vi "IMAQController.destructor.vi"(0 "i ref in":refnum<vi>, 5 "error in (no error)":errorcluster) -> (19 "error out":errorcluster)   [LabVIEW 2014, in "IMAQController.lvlib"]
doc: "This is the destructor of a class.\n\nLicense Agreement for this software:\n\nCopyright (C)\nGesellschaft für Schwerionenforschung, GSI\nPlanckstr. 1\n64291 Darmstadt\nGermany\n\nContact: D.Beck@gsi.de \n\nThis program is free software; you can redistribute it and/or modify it under the terms of the \nGNU General Public License as published by the Free Software Foundation; either version 2 of \nthe license, or (at your option) any later version.\n\nThis program is distributed in the hope that it will be useful, but WITHOUT ANY WARRANTY; \nwithout even the implied warranty of MERCHANTABILITY or FITNESS FOR A PARTICULAR PURPOSE. See the GNU General License for more details (http://www.gnu.org).\n\nGesellschaft für Schwerionenforschung, GSI\nPlanckstr. 1, 64291 Darmstadt, Germany\nFor all questions and ideas contact: M.Richter@gsi.de, H.Brand@gsi.de or D.Beck@gsi.de.\nLast update: 16-JUN-2004"
uses:
  IMAQController.lvlib
  CSCore/CSSystem/CoreLib/CoreLib.string 2 byte array.vi
  CSCore/BaseGUI/BaseGUI.lvlib
  CSCore/BaseProcess/BaseProcess.lvlib
  CSlibraries-extern/DimLVEvent/LVDimInterface/LVDimInterface.lvlib
  CSCore/CSSystem/CSSystemLib/CSSystemLib.lvlib
  CSCore/CSSystem/CoreLib/CoreLib.lvlib
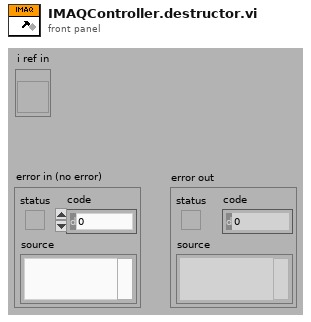
[diagram p1: front panel]
types:
  T1 = typedef "IMAQController.lvlib/IMAQController.i attribute.ctl" = cluster{"ImageTakenID":i32, "actSequencer":string, "actScanner":string, "CameraTriggerID":i32, "activatedCameras":cluster{"Name":string, "Camera Type":string, "Acquisition Mode":u32, "JPEG Mode?":bool, "Acquisition Delay":dbl, "Save Images?":bool, "Center Coordinates":T2, "PixelPermm":cluster{"Horizontal":dbl, "Vertical":dbl}, "Rotation":dbl, "Mirror Mode":u32, "PixelCoordinates":cluster{"1":cluster{"Horizontal":i32, "Vertical":i32}, "2":cluster{"Horizontal":i32, "Vertical":i32}, "3":cluster{"Horizontal":i32, "Vertical":i32}, "4":cluster{"Horizontal":i32, "Vertical":i32}}, "RWCoordinates":cluster{"1":cluster{"Horizontal":dbl, "Vertical":dbl}, "2":cluster{"Horizontal":dbl, "Vertical":dbl}, "3":cluster{"Horizontal":dbl, "Vertical":dbl}, "4":cluster{"Horizontal":dbl, "Vertical":dbl}}, "HorizScaling":dbl, "VertScaling":dbl}[], "Ini C-Array":string[], "actCamera":string, "activeCamera":cluster{"Name":string, "Camera Type":string, "Aqcuisation Mode":enum32{"Internal Trigger", "Scan", "free Running", "External Trigger"}, "JPEG Mode?":bool, "Acquisition Delay":dbl, "Save Images?":bool, "Center Coordinates":T2, "PixelPermm":cluster{"Horizontal":dbl, "Vertical":dbl}, "Rotation":dbl, "Mirror Mode":u32, "PixelCoordinates":cluster{"1":cluster{"Horizontal":i32, "Vertical":i32}, "2":cluster{"Horizontal":i32, "Vertical":i32}, "3":cluster{"Horizontal":i32, "Vertical":i32}, "4":cluster{"Horizontal":i32, "Vertical":i32}}, "RWCoordinates":cluster{"1":cluster{"Horizontal":dbl, "Vertical":dbl}, "2":cluster{"Horizontal":dbl, "Vertical":dbl}, "3":cluster{"Horizontal":dbl, "Vertical":dbl}, "4":cluster{"Horizontal":dbl, "Vertical":dbl}}, "HorizScaling":dbl, "VertScaling":dbl}, "BilderMittelungen":u8, "OldPicture":dbl[][]}
  T2 = typedef "LVPoint32TypeDef.ctl" = cluster{"Horizontal":i32, "Vertical":i32}
  T3 = enum16{"SetAttribute", "GetAttribute", "CreateAttribute", "DestroyAttribute", "DestroyAllAtributes"}
  T4 = typedef "CoreDefs.rawDataType.ctl" = i8[]
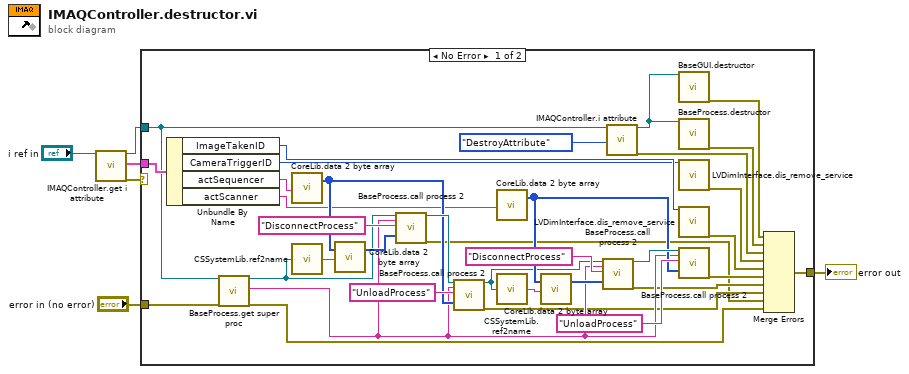
[diagram p0: block diagram]
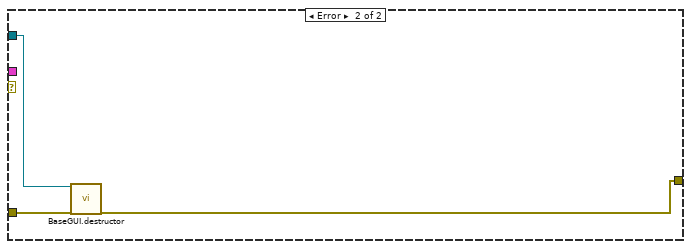
[diagram p2: hidden frame]
diagram:
  n1 = call "IMAQController.get i attribute.vi"("i ref in"="i ref in") -> ("i ref out"=w3:refnum<vi>, "i attribute"=w1:T1, "error out"=w2:errorcluster)  [unwired: 16 in]
  n2 = case shown="No Error" w2 {
    tunnel: [w7 w42] -> w6
    tunnel: w3 -> [w30 w44]
    tunnel: "error in (no error)" -> [w29 w43]
    tunnel: w1 -> [w39 _]
    frame No Error {
      n3 = Unbundle By Name(w39) -> ("ImageTakenID"=w38:i32, "CameraTriggerID"=w37:i32, "actSequencer"=w27:string, "actScanner"=w19:string)
      n4 = call "BaseProcess.get super proc.vi"("i ref in"=w30, "error in (no error)"=w29) -> ("i ref out"=w28:refnum<vi>, "SuperProc"=w20:string, "error out"=w8:errorcluster)  [unwired: 15 in]
      n5 = call-poly "CoreLib.data 2 byte array.vi"("string"=w27) -> ("byteArray out"=w31:T4)  [unwired: 18 in]
      n6 = call "CSSystemLib.ref2name.vi"("obj refnum"=w28) -> ("name"=w35:string)
      n7 = call-poly "CoreLib.data 2 byte array.vi"("byteArray"=w31, "string"=w35) -> ("byteArray out"=w34:T4)  [unwired: 17 in]
      n8 = call "BaseProcess.call process 2.vi"("i ref in"=w28, "Object"=w20, "Selector"="DisconnectProcess", "Data"=w34) -> ("i ref out"=w33:refnum<vi>, "error out"=w9:errorcluster)  [unwired: 14 in]
      n9 = call "BaseProcess.call process 2.vi"("i ref in"=w33, "Object"=w20, "Selector"="UnloadProcess", "Data"=w31) -> ("i ref out"=w18:refnum<vi>, "error out"=w10:errorcluster)  [unwired: 14 in]
      n10 = call-poly "CoreLib.data 2 byte array.vi"("string"=w19) -> ("byteArray out"=w21:T4)  [unwired: 18 in]
      n11 = call "CSSystemLib.ref2name.vi"("obj refnum"=w18) -> ("name"=w25:string)
      n12 = call-poly "CoreLib.data 2 byte array.vi"("byteArray"=w21, "string"=w25) -> ("byteArray out"=w24:T4)  [unwired: 17 in]
      n13 = call "BaseProcess.call process 2.vi"("i ref in"=w18, "Object"=w20, "Selector"="DisconnectProcess", "Data"=w24) -> ("i ref out"=w23:refnum<vi>, "error out"=w11:errorcluster)  [unwired: 14 in]
      n14 = call "IMAQController.i attribute.vi"("VI Refnum"=w30, "Action"=T3."DestroyAttribute") -> ("VI Refnum out"=w40:refnum<vi>, "error out"=w15:errorcluster)  [unwired: 15 in, 1 out]
      n15 = call "BaseGUI.destructor.vi"("i ref in"=w40) -> ("error out"=w17:errorcluster)  [unwired: 18 in]
      n16 = call "BaseProcess.destructor.vi"("i ref in"=w40) -> ("error out"=w16:errorcluster)  [unwired: 18 in]
      n17 = call "LVDimInterface.dis_remove_service.vi"("my_serviceID"=w37) -> ("error out"=w14:errorcluster)  [unwired: 18 in]
      n18 = call "LVDimInterface.dis_remove_service.vi"("my_serviceID"=w38) -> ("error out"=w13:errorcluster)  [unwired: 18 in]
      n19 = call "BaseProcess.call process 2.vi"("i ref in"=w23, "Object"=w20, "Selector"="UnloadProcess", "Data"=w21) -> ("error out"=w12:errorcluster)  [unwired: 14 in, 1 out]
      n20 = Merge Errors(w17, w16, w15, w14, w13, w12, w11, w10, w9, w8) -> (w7:errorcluster)
    }
    frame Error {
      n21 = call "BaseGUI.destructor.vi"("i ref in"=w44, "error in (no error)"=w43) -> ("error out"=w42:errorcluster)  [unwired: 17 in]
    }
  }
  "error out" <- w6
